vi "integrated_syringe_motor.vi"() -> ()   [LabVIEW 2014]
uses:
  <vilib>/Motion/FlexMotion/CustomControls/CustomControls.llb/AxisOrVectorSpace To Configure.flx
  <vilib>/Motion/FlexMotion/FunctionsVIs/StartStopMotion.llb/Start Motion (8 axes).flx
  <vilib>/Motion/FlexMotion/FunctionsVIs/Trajectory.llb/Check Move Complete Status (8 axes).flx
  <vilib>/Motion/FlexMotion/FunctionsVIs/StartStopMotion.llb/Stop Motion (8 axes).flx
  <instrlib>/KD Scientific 2XX Series/KD Scientific 2XX Series.lvlib
panel:
  out "Status":T1
  in  "stop":bool
  out "Delivered Volume":dbl
  out "Units":string
  in  "Flow Rate (5)":dbl=5.0
  in  "Units (0: milliliters)":u16(ring) items=["milliliters (ml)", "microliters (ul)"]
  in  "Volume (100)":dbl=100.0
  in  "Diameter (8.75 mm)":dbl=8.75
  in  "Mode (infuse)":u16(ring) items=["Infuse", "Withdraw", "Infuse-Withdraw", "Withdraw-Infuse", "Continuous"]
  in  "Address (0)":i32
  in  "error in (no error)":errorcluster
  in  "Baud Rate (9600)":u32(ring)=9600 items=["300"=300, "1200"=1200, "2400"=2400, "4800"=4800, "9600"=9600]
  in  "VISA resource name":refnum<visa-resource-name>
  in  "Velocity (10000)":i32=10000 min=-20000000 max=20000000
  in  "Target Position (0)":i32
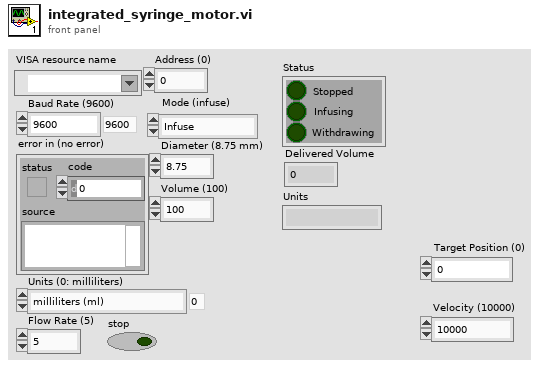
[diagram p1: front panel]
types:
  T1 = cluster{"Stopped":bool, "Infusing":bool, "Withdrawing":bool}
  T2 = typedef "Board Id" = u8
  T3 = enum16{"Absolute Position", "Relative Position", "Velocity", "Relative to Cap Pos", "Modulus Position", "Absolute Contouring", "Relative Contouring"}
  T4 = typedef "AxisOrVectorSpace To Configure.flx" = u16
  T5 = typedef "Resource Out (Enum).flx" = u16
  T6 = typedef "Bd Id Out" = u8
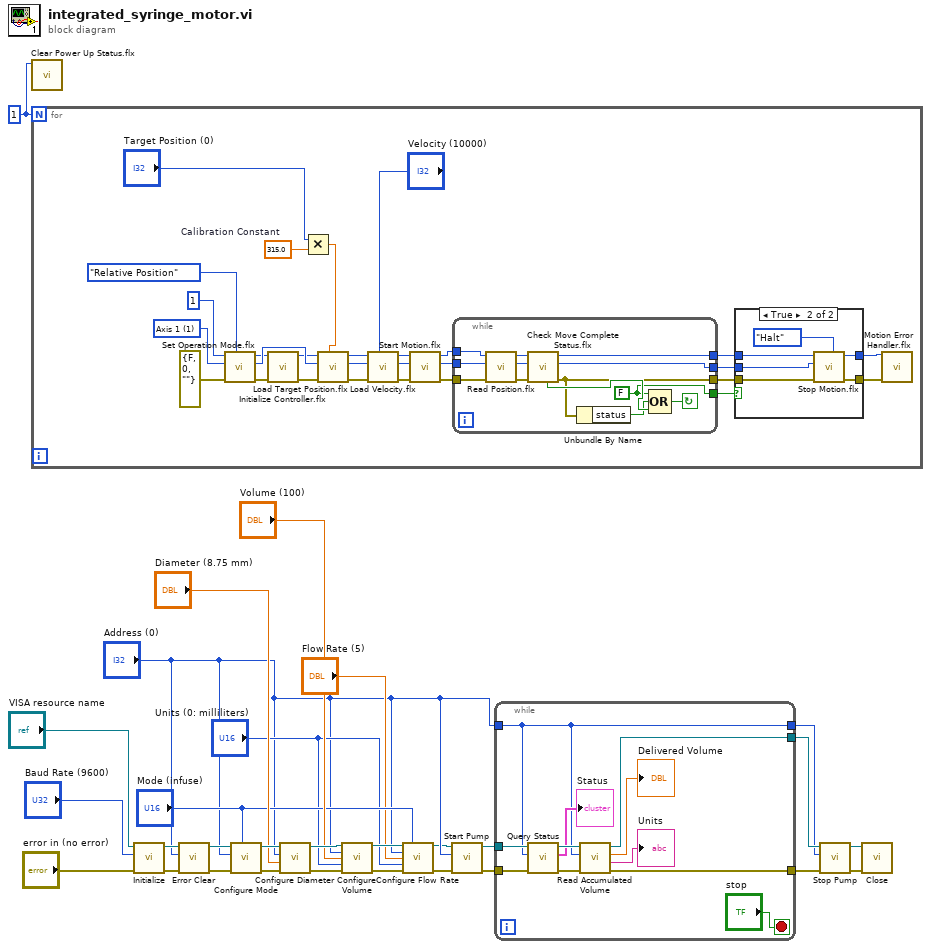
[diagram p0: block diagram]
diagram:
  w29 = T2 1 ("Board ID")
  n1 = call <vilib>:"Clear Power Up Status.flx"("Board ID"=w29) -> ()  [unwired: 6 in, 2 out]
  n2 = for {
    N: w29 -> [_]
    w32 = 315.0  # Calibration Constant
    w55 = T4 1 items=["Axis 1"=1, "Axis 2"=2, "Axis 3"=3, "Axis 4"=4, "Axis 5"=5, "Axis 6"=6, "Axis 7"=7, "Axis 8"=8, "Vector Space 1"=17, "Vector Space 2"=18, "Vector Space 3"=19, "Vector Space 4"=20] ("Axis or Vector Space")
    n3 = call <vilib>:"Set Operation Mode.flx"("Position Mode (Absolute)"=T3."Relative Position", "error in (no error)"=errorcluster {"status"=FALSE, "code"=0, "source"=""} ("error constant"), "Axis or Vector Space"=w55, "Board ID"=T2 1) -> ("error out"=w53:errorcluster, "Resource Output"=w52:T5, "Bd ID Out"=w51:T6)  [unwired: 2 in]
    n4 = call <vilib>:"Initialize Controller.flx"("error in (no error)"=w53, "Board ID"=w51) -> ("error out"=w46:errorcluster, "Bd ID Out"=w50:T6)  [unwired: 6 in]
    n5 = Multiply(x="Target Position (0)", y=w32) -> (x*y=w30:dbl)
    n6 = call <vilib>:"Load Target Position.flx"("Target Position (0)"=w30, "error in (no error)"=w46, "Axis"=w52, "Board ID"=w50) -> ("error out"=w47:errorcluster, "Resource Output"=w48:T5, "Bd ID Out"=w49:T6)  [unwired: 3 in]
    n7 = call <vilib>:"Load Velocity.flx"("Velocity (10000)"="Velocity (10000)", "error in (no error)"=w47, "Axis or Vector Space"=w48, "Board ID"=w49) -> ("error out"=w43:errorcluster, "Resource Output"=w44:T5, "Bd ID Out"=w45:T6)  [unwired: 3 in]
    n8 = call-poly <vilib>:"Start Motion.flx"("error in (no error)"=w43, "Axis or Vector Space"=w44, "Board ID"=w45) -> ("error out"=w40:errorcluster, "Resource Output"=w41:T5, "Bd ID Out"=w42:T6)  [unwired: 3 in]
    n9 = while {
      tunnel: w42 -> [w78]
      tunnel: w41 -> [w77]
      tunnel: w40 -> [w76]
      tunnel: [w70] -> w39
      tunnel: [w69] -> w38
      tunnel: [w67] -> w37
      tunnel: [w66] -> w36
      stop <- w71 continue-if-true
      w70 = FALSE
      n10 = call <vilib>:"Read Position.flx"("error in (no error)"=w76, "Axis"=w77, "Board ID"=w78) -> ("error out"=w73:errorcluster, "Resource Output"=w74:T5, "Bd ID Out"=w75:T6)  [unwired: 3 in, 1 out]
      n11 = call-poly <vilib>:"Check Move Complete Status.flx"("error in (no error)"=w73, "Axis or Vector Space"=w74, "Board ID"=w75) -> ("error out"=w69:errorcluster, "Resource Output"=w66:T5, "Bd ID Out"=w67:T6, "Move Complete"=w72:bool)  [unwired: 3 in]
      n12 = Unbundle By Name(w69) -> ("status"=w68:bool)
      n13 = Compound Arithmetic op=OR(w70, w68, w72) -> (w71:bool)
    }
    n14 = case shown="True" w39 {
      tunnel: w38 -> [w58 w64]
      tunnel: w37 -> [w59 w63]
      tunnel: w36 -> [_ w62]
      tunnel: [w58 w61] -> w35
      tunnel: [w59 w60] -> w34
      frame False {
      }
      frame True {
        n15 = call-poly <vilib>:"Stop Motion.flx"("Stop Type (Decel)"=enum16{"Decelerate", "Halt", "Kill"}."Halt", "error in (no error)"=w64, "Axis or Vector Space"=w62, "Board ID"=w63) -> ("error out"=w61:errorcluster, "Bd ID Out"=w60:T6)  [unwired: 3 in, 1 out]
      }
    }
    n16 = call <vilib>:"Motion Error Handler.flx"("Board ID"=w34, "error in (no error)"=w35) -> ()  [unwired: 9 in, 5 out]
  }
  n17 = call <instrlib>:"Initialize.vi"("error in (no error)"="error in (no error)", "Baud Rate (9600)"="Baud Rate (9600)", "VISA resource name"="VISA resource name") -> ("error out"=w24:errorcluster, "VISA resource name out"=w25:refnum<visa-resource-name>)  [unwired: 7 in]
  n18 = call <instrlib>:"Error Clear.vi"("error in (no error)"=w24, "Address (0)"="Address (0)", "VISA resource name"=w25) -> ("error out"=w22:errorcluster, "VISA resource name out"=w23:refnum<visa-resource-name>)  [unwired: 6 in, 1 out]
  n19 = call <instrlib>:"Configure Mode.vi"("Mode (infuse)"="Mode (infuse)", "error in (no error)"=w22, "Address (0)"="Address (0)", "VISA resource name"=w23) -> ("error out"=w13:errorcluster, "VISA resource name out"=w14:refnum<visa-resource-name>)  [unwired: 6 in]
  n20 = call <instrlib>:"Configure Diameter.vi"("error in (no error)"=w13, "Diameter (8.75 mm)"="Diameter (8.75 mm)", "Address (0)"="Address (0)", "VISA resource name"=w14) -> ("error out"=w10:errorcluster, "VISA resource name out"=w11:refnum<visa-resource-name>)  [unwired: 6 in]
  n21 = call <instrlib>:"Configure Volume.vi"("VISA resource name"=w11, "Address (0)"="Address (0)", "Volume (100)"="Volume (100)", "Units (0: milliliters)"="Units (0: milliliters)", "error in (no error)"=w10) -> ("VISA resource name out"=w8:refnum<visa-resource-name>, "error out"=w7:errorcluster)  [unwired: 9 in]
  n22 = call <instrlib>:"Configure Flow Rate.vi"("VISA resource name"=w8, "Mode (infuse)"="Mode (infuse)", "Address (0)"="Address (0)", "Flow Rate (5)"="Flow Rate (5)", "Units (0: milliliters per minute)"="Units (0: milliliters)", "error in (no error)"=w7) -> ("VISA resource name out"=w2:refnum<visa-resource-name>, "error out"=w1:errorcluster)  [unwired: 8 in]
  n23 = call <instrlib>:"Start Pump.vi"("error in (no error)"=w1, "Address (0)"="Address (0)", "VISA resource name"=w2) -> ("error out"=w20:errorcluster, "VISA resource name out"=w21:refnum<visa-resource-name>)  [unwired: 7 in]
  n24 = while {
    tunnel: w21 -> [w89]
    tunnel: w20 -> [w88]
    tunnel: "Address (0)" -> [w80]
    tunnel: [w82] -> w19
    tunnel: [w81] -> w18
    tunnel: [w80] -> w17
    stop <- "stop" stop-if-true
    n25 = call <instrlib>:"Query Status.vi"("error in (no error)"=w88, "Address (0)"=w80, "VISA resource name"=w89) -> ("error out"=w86:errorcluster, "Status"=→"Status":T1, "VISA resource name out"=w87:refnum<visa-resource-name>)  [unwired: 6 in]
    n26 = call <instrlib>:"Read Accumulated Volume.vi"("error in (no error)"=w86, "Address (0)"=w80, "VISA resource name"=w87) -> ("error out"=w81:errorcluster, "Units"=→"Units":string, "Delivered Volume"=→"Delivered Volume":dbl, "VISA resource name out"=w82:refnum<visa-resource-name>)  [unwired: 5 in]
  }
  n27 = call <instrlib>:"Stop Pump.vi"("error in (no error)"=w18, "Address (0)"=w17, "VISA resource name"=w19) -> ("error out"=w15:errorcluster, "VISA resource name out"=w16:refnum<visa-resource-name>)  [unwired: 7 in]
  n28 = call <instrlib>:"Close.vi"("error in (no error)"=w15, "VISA resource name"=w16) -> ()  [unwired: 9 in, 1 out]
